vi "DriveSystemMode.vi"() -> ()   [LabVIEW 2012]
uses:
  Controls/Drive System Mode.ctl
panel:
  in  "Drive System Mode":T1
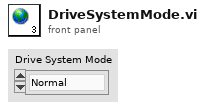
[diagram p1: front panel]
types:
  T1 = typedef "Drive System Mode.ctl" = enum16{"Normal", "Crab", "Shoot"}
diagram:
